vi "Control_Test.vi"() -> ()   [LabVIEW 2020]
uses:
  States.ctl
  <vilib>/Utility/file.llb/Read Delimited Spreadsheet (I64).vi
panel:
  out "First State":T1
  out "error constant":errorcluster
  out "Time Left":u32
  out "Inc Changed":bool
  out "Next MPH":u16
  out "Next Duration":u16
  out "Next Inc":u16
  out "dwell":u16[](array[numeric])
  out "incline":u16[](array[numeric])
  out "time":u16[](array[numeric])
  out "speed":u16[](array[numeric])
  out "input lines":i32
  in  "TestScript":path=path "C:/LabView Computer Backup SEAL2788/DonP_TRM500/FootTimeInc.txt"
  out "Speed Changed":bool
  out "stopping":bool
  out "Target MPH":u16 max=12 step=1
  out "step":i32
  out "INC":u16 max=12 step=1
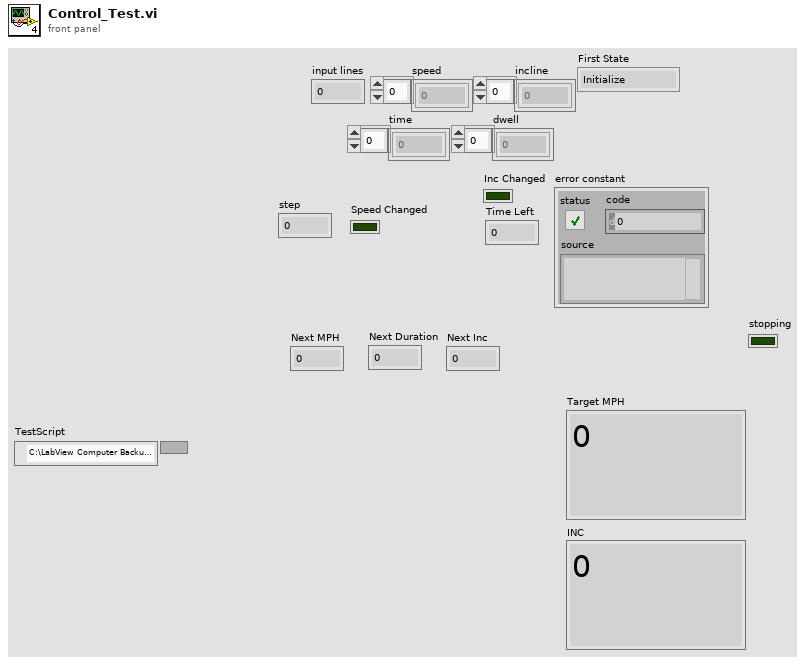
[diagram p1: front panel]
types:
  T1 = typedef "States.ctl" = enum16{"Initialize", "SetTargets", "WaitforMPH", "Dwell", "CheckTiming"}
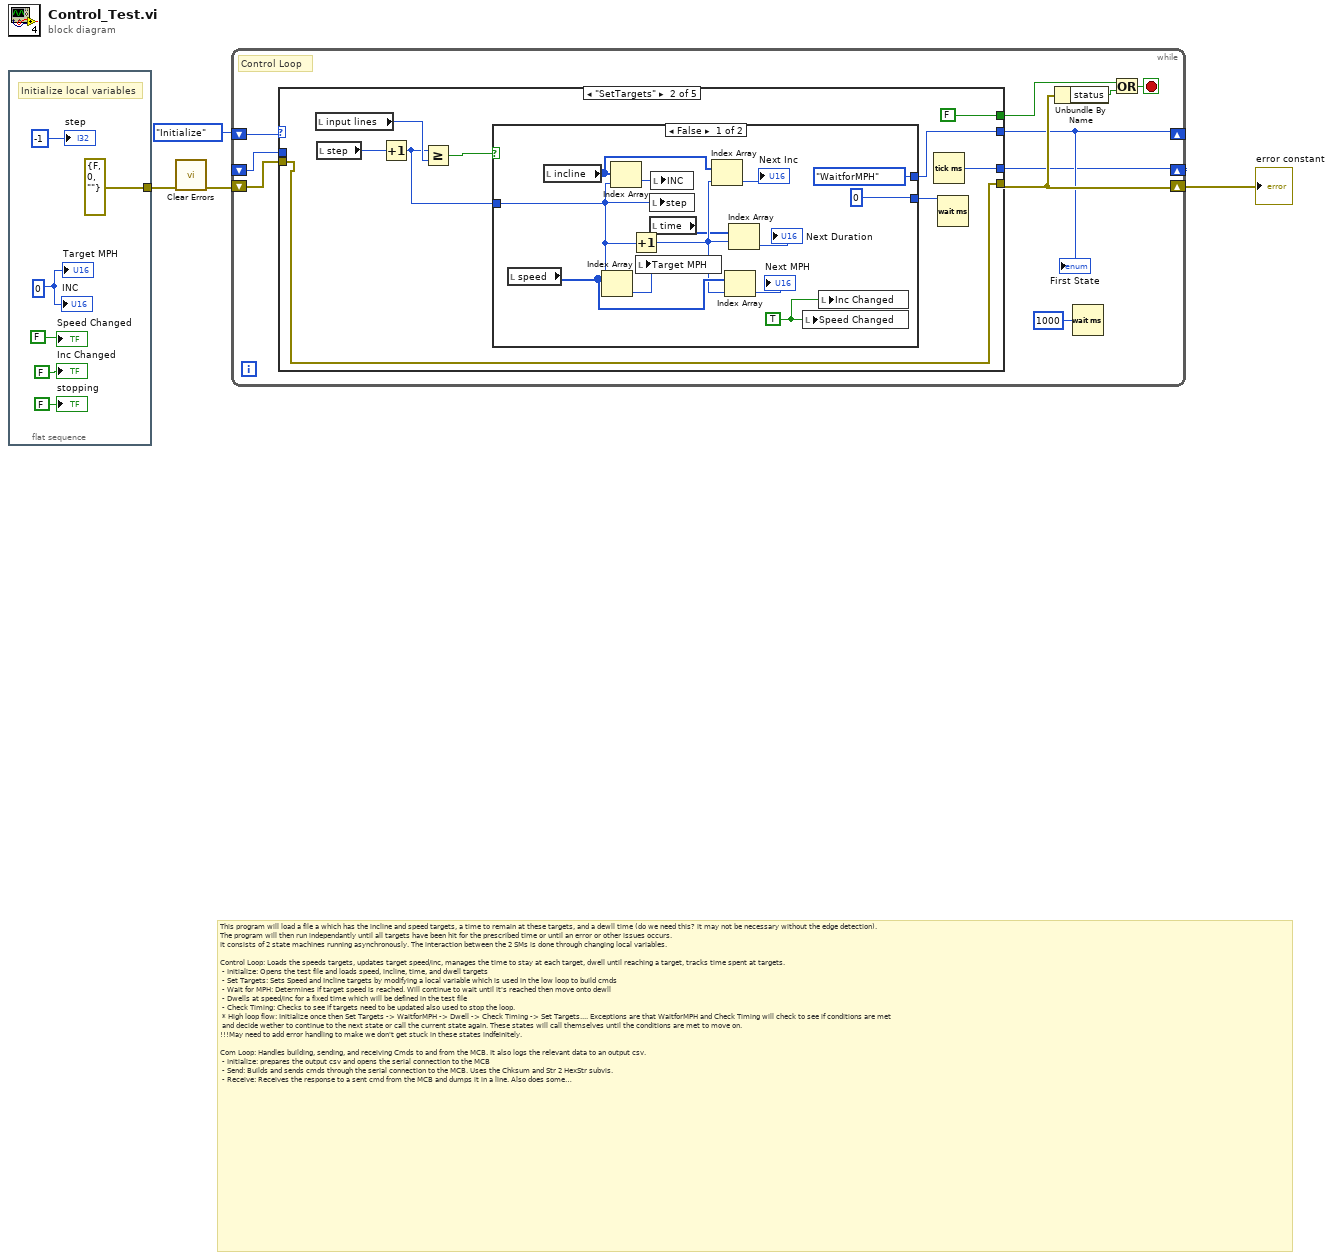
[diagram p0: block diagram]
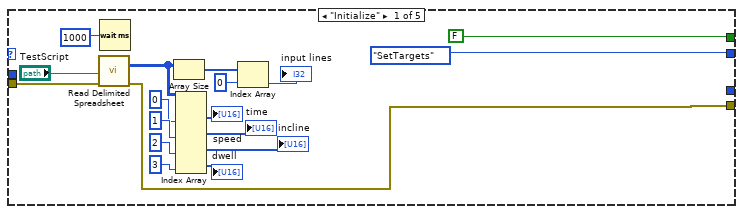
[diagram p2: hidden frame]
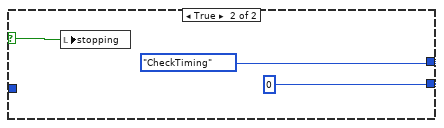
[diagram p3: hidden frame]
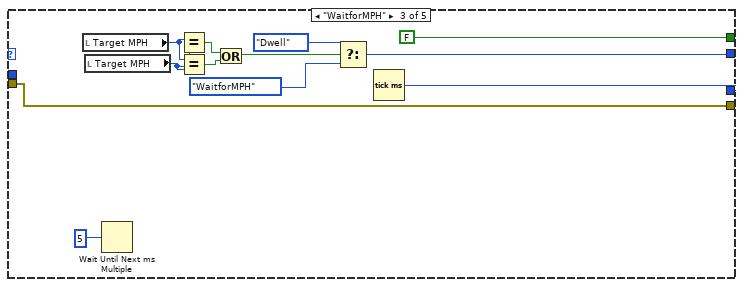
[diagram p4: hidden frame]
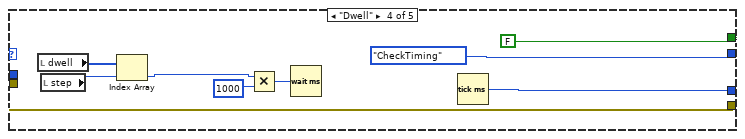
[diagram p5: hidden frame]
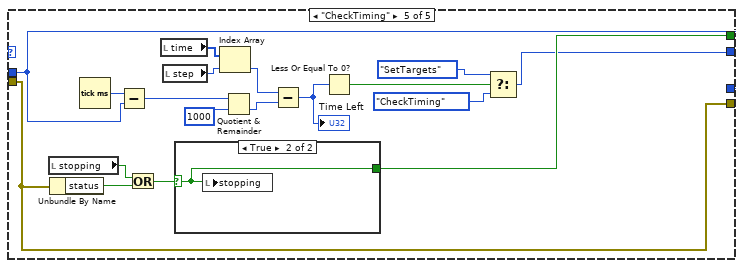
[diagram p6: hidden frame]
diagram:
  # "This program will load a file a which has the incline and speed targets, a time to remain at these targets, and a dewll time (do we need this? it may not be necessary without the edge detection).\nThe program will then run independantly until all targets have been hit for the prescribed time or until an error or other issues occurs.\nIt consists of 2 state machines running asynchronously. The interaction between the 2 SMs is done through changing local variables.\n\nControl Loop: Loads the speeds targets, updates target speed/inc, manages the time to stay at each target, dwell until reaching a target, tracks time spent at targets. \n - Initialize: Opens the test file and loads speed, incline, time, and dwell targets \n - Set Targets: Sets Speed and Incline targets by modifying a local variable which is used in the low loop to build cmds \n - Wait for MPH: Determines if target speed is reached. Will continue to wait until it's reached then move onto dewll\n - Dwells at speed/inc for a fixed time which will be defined in the test file\n - Check Timing: Checks to see if targets need to be updated also used to stop the loop.\n * High loop flow: Initialize once then Set Targets -> WaitforMPH -> Dwell -> Check Timing -> Set Targets.... Exceptions are that WaitforMPH and Check Timing will check to see if conditions are met\n and decide wether to continue to the next state or call the current state again. These states will call themselves until the conditions are met to move on. \n!!!May need to add error handling to make we don't get stuck in these states indfeinitely.\n\nCom Loop: Handles building, sending, and receiving Cmds to and from the MCB. It also logs the relevant data to an output csv.\n - Initialize: prepares the output csv and opens the serial connection to the MCB\n - Send: Builds and sends cmds through the serial connection to the MCB. Uses the Chksum and Str 2 HexStr subvis. \n - Receive: Receives the response to a sent cmd from the MCB and dumps it in a line. Also does some analysis of the response to determine current  Speed/inc/person detect\n - Error:  Stops the program. This handles labview errors and will stop the program when one is encounted. It also handles stopping when reaching the end of a test \n * Low loop flow: nitialize once then Send -> Receive -> Error -> Send...\n * Send flow: GetParm -> Inc -> MPH -> GetParm etc. Exception is that it will check first to see if the target changed and if it hasn't will send getParm Instead\n  !!!May need to add error handling in which case the flow should be GetParm -> MPH -> Inc -> Err -> GetParm...."
  n1 = flat-sequence {
    tunnel: [errorcluster {"status"=FALSE, "code"=0, "source"=""} ("error constant")] -> w3
    frame #0 {
      w6 = u16 0 ("MPH")
      # "Initialize local variables"
      "stopping" <- FALSE ("stopping")
      "Target MPH" <- w6
      "step" <- -1 ("step")
      "INC" <- w6
      "Speed Changed" <- FALSE ("Value Changed")
      "Inc Changed" <- FALSE ("Inc Changed")
    }
  }
  n2 = call <vilib>:"Clear Errors.vi"("error in (no error)"=w3) -> ("error out"=w2:errorcluster)  [unwired: 5 in, 1 out]
  n3 = while {
    shift-right: [w16] -> w4
    shift-left: w2 -> [w20]
    shift-right: [w14] -> _
    shift-left: _ -> [w13]
    shift-right: [w15] -> _
    shift-left: States."Initialize" ("First State") -> [w12]
    stop <- w18 stop-if-true
    # "Control Loop"
    n4 = case shown="\"SetTargets\"" w12 {
      tunnel: w20 -> [w36 w39 w74 w81 w85]
      tunnel: [FALSE FALSE FALSE FALSE w98] -> w17
      tunnel: [w25 w39 w74 w81 w85] -> w16
      tunnel: [States."SetTargets" ("First State") w44 w71 States."CheckTiming" ("First State") w86] -> w15
      tunnel: [_ w41 w72 w78 w97] -> w14
      tunnel: w13 -> [_ _ _ _ w97]
      frame "Initialize" {
        n5 = call-poly <vilib>:"Read Delimited Spreadsheet.vi"("file path (dialog if empty)"="TestScript", "error in (no error)"=w36) -> ("all rows"=w32:i64[][], "error out"=w25:errorcluster)  [unwired: 8 in, 4 out]
        n6 = Wait (ms)(milliseconds to wait=u32 1000) -> ()  [unwired: 1 out]
        n7 = Array Size(array=w32) -> (size(s)=w34:i32[])
        n8 = Index Array(array=w32, index (col) #1=0 ("index"), index (col) #2=1 ("index (col)"), index (col) #3=2 ("index (col)"), index (col) #4=3 ("index (col)")) -> (element #1=→"speed":i64[], element #2=→"time":i64[], element #3=→"incline":i64[], element #4=→"dwell":i64[])  [unwired: 4 in]
        n9 = Index Array(array=w34, index=0) -> (element=→"input lines":i32)
      }
      frame "SetTargets" {
        n10 = local read "input lines"() -> (w46:i32)
        n11 = local read "step"() -> (w47:i32)
        n12 = Increment(x=w47) -> (x+1=w40:i32)
        n13 = Greater Or Equal?(x=w40, y=w46) -> (x >= y?=w45:bool)
        n14 = case shown="False" w45 {
          selector: w45 -> [_ w63]
          tunnel: [States."WaitforMPH" ("First State") States."CheckTiming" ("First State")] -> w44
          tunnel: [u32 0 ("milliseconds to wait") u32 0 ("milliseconds to wait")] -> w43
          tunnel: w40 -> [w58 _]
          frame False {
            w49 = TRUE ("Value Changed")
            n15 = local read "speed"() -> (w57:u16[])
            n16 = local read "incline"() -> (w56:u16[])
            n17 = Index Array(array=w57, index=w58) -> (element=w60:u16)
            n18 = Index Array(array=w56, index=w58) -> (element=w59:u16)
            n19 = Increment(x=w58) -> (x+1=w55:i32)
            n20 = local write "Target MPH"(w60) -> ()
            n21 = local write "step"(w58) -> ()
            n22 = local read "time"() -> (w54:u16[])
            n23 = local write "INC"(w59) -> ()
            n24 = Index Array(array=w56, index=w55) -> (element=→"Next Inc":u16)
            n25 = Index Array(array=w57, index=w55) -> (element=→"Next MPH":u16)
            n26 = Index Array(array=w54, index=w55) -> (element=→"Next Duration":u16)
            n27 = local write "Speed Changed"(w49) -> ()
            n28 = local write "Inc Changed"(w49) -> ()
          }
          frame True {
            n29 = local write "stopping"(w63) -> ()
          }
        }
        n30 = Tick Count (ms)() -> (millisecond timer value=w41:u32)
        n31 = Wait (ms)(milliseconds to wait=w43) -> ()  [unwired: 1 out]
      }
      frame "WaitforMPH" {
        n32 = local read "Target MPH"() -> (w67:u16)
        n33 = local read "Target MPH"() -> (w64:u16)
        n34 = Wait Until Next ms Multiple(millisecond multiple=u32 5) -> ()  [unwired: 1 out]
        n35 = Equal?(x=w67, y=w64) -> (x = y?=w69:bool)
        n36 = Equal?(x=w67, y=w64) -> (x = y?=w68:bool)
        n37 = Or(x=w69, y=w68) -> (x .or. y?=w70:bool)
        n38 = Select(t=States."Dwell" ("First State"), s=w70, f=States."WaitforMPH" ("First State")) -> (s? t:f=w71:T1)
        n39 = Tick Count (ms)() -> (millisecond timer value=w72:u32)
      }
      frame "Dwell" {
        n40 = local read "dwell"() -> (w79:u16[])
        n41 = local read "step"() -> (w80:i32)
        n42 = Index Array(array=w79, index=w80) -> (element=w84:u16)
        n43 = Multiply(x=w84, y=u16 1000) -> (x*y=w82:u16)
        n44 = Wait (ms)(milliseconds to wait=w82) -> ()  [unwired: 1 out]
        n45 = Tick Count (ms)() -> (millisecond timer value=w78:u32)
      }
      frame "CheckTiming" {
        n46 = local read "stopping"() -> (w100:bool)
        n47 = Unbundle By Name(w85) -> ("status"=w101:bool)
        n48 = Tick Count (ms)() -> (millisecond timer value=w102:u32)
        n49 = Subtract(x=w102, y=w97) -> (x-y=w96:u32)
        n50 = Or(x=w100, y=w101) -> (x .or. y?=w99:bool)
        n51 = local read "time"() -> (w94:u16[])
        n52 = local read "step"() -> (w93:i32)
        n53 = case shown="True" w99 {
          selector: w99 -> [w103 w104]
          tunnel: [w103 w104] -> w98
          frame False {
          }
          frame True {
            n54 = local write "stopping"(w104) -> ()
          }
        }
        n55 = Index Array(array=w94, index=w93) -> (element=w91:u16)
        n56 = Quotient & Remainder(x=w96, y=u32 1000) -> (floor(x/y)=w92:u32)  [unwired: 1 out]
        n57 = Subtract(x=w91, y=w92) -> (x-y=w90:u32)
        "Time Left" <- w90
        n58 = Less Or Equal To 0?(x=w90) -> (x <= 0?=w89:bool)
        n59 = Select(t=States."SetTargets" ("First State"), s=w89, f=States."CheckTiming" ("First State")) -> (s? t:f=w86:T1)
      }
    }
    "First State" <- w15
    n60 = Unbundle By Name(w16) -> ("status"=w19:bool)
    n61 = Wait (ms)(milliseconds to wait=u32 1000) -> ()  [unwired: 1 out]
    n62 = Or(x=w17, y=w19) -> (x .or. y?=w18:bool)
  }
  "error constant" <- w4
